vi "AbortReachGoal_set.vi"(8 "error in (no error)":errorcluster, 10 "Abort? (F)":bool) -> (0 "error out":errorcluster)   [LabVIEW 2009, in "Main.lvlib" / "MainVariables.lvlib"]
doc: "Set value of AbortReachGoal variable"
uses:
  MainVariables.lvlib
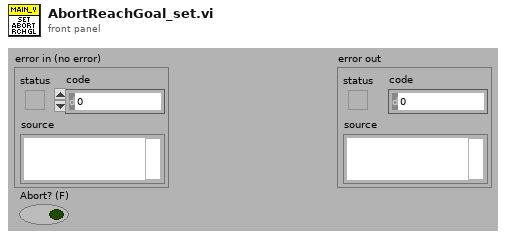
[diagram p1: front panel]
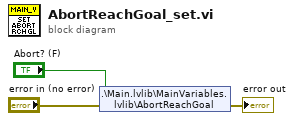
[diagram p0: block diagram]
diagram:
  n1 = shared-variable ".\\Main.lvlib\\MainVariables.lvlib\\AbortReachGoal"("Abort? (F)", error in="error in (no error)") -> (error out=→"error out":errorcluster)
